vi "Content.vi"(7 "Context":refnum<class "Context.lvclass">, 8 "Error In":errorcluster, 11 "Tag In":refnum<class "Tag.lvclass">) -> (0 "Error Out":errorcluster, 2 "Content":string, 3 "Tag Out":refnum<class "Tag.lvclass">)   [LabVIEW 2018, in "Toolkit.lvlib" / "Nodes.lvlib" / "Tag.lvclass"]
uses:
  Tag.lvclass
  Support/Context/Context.lvclass
  Tag.lvclass/Tag.ctl
  Data/String/String.lvclass
  Data/String/String.lvclass/String.ctl
  Data/Abstract/Abstract.lvclass
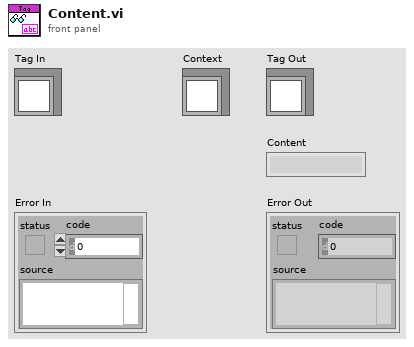
[diagram p1: front panel]
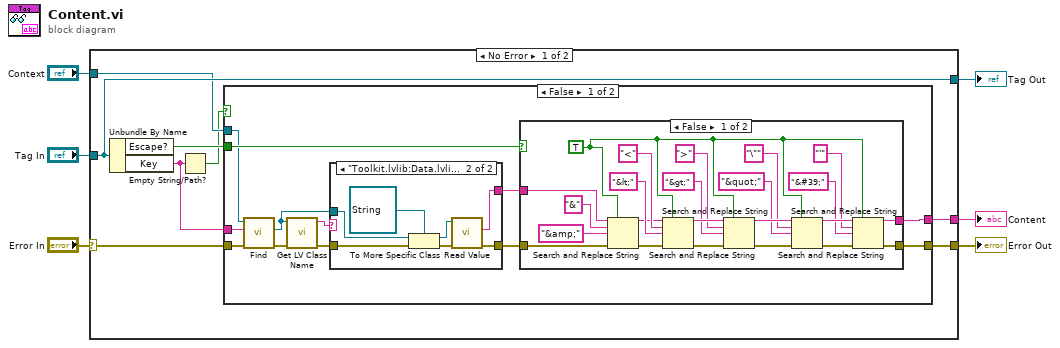
[diagram p0: block diagram]
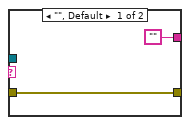
[diagram p2: hidden frame]
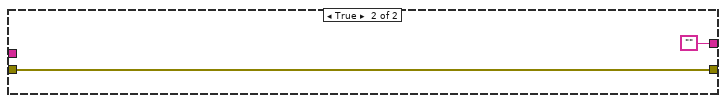
[diagram p4: hidden frame]
diagram:
  n1 = case shown="No Error" "Error In" {
    selector: "Error In" -> [w9 w63]
    tunnel: "Tag In" -> [w14 w64]
    tunnel: [w14 w64] -> w4
    tunnel: [w13 w63] -> w3
    tunnel: [w12 _] -> w2
    tunnel: "Context" -> [w10 _]
    frame No Error {
      n2 = Unbundle By Name(w14) -> ("Escape?"=w11:bool, "Key"=w8:string)
      n3 = Empty String/Path?(string/path=w8) -> (empty?=w7:bool)
      n4 = case shown="False" w7 {
        tunnel: [w26 w62] -> w13
        tunnel: [w25 ""] -> w12
        tunnel: w11 -> [w24 _]
        tunnel: w10 -> [w19 _]
        tunnel: w8 -> [w18 _]
        tunnel: w9 -> [w17 w62]
        frame False {
          n5 = call "Find.vi"("Error In"=w17, "Key"=w18, "Context In"=w19) -> ("Error Out"=w16:errorcluster, "Datum"=w15:refnum<class "Abstract.lvclass">)  [unwired: 5 in, 2 out]
          n6 = call <vilib>:"Get LV Class Name.vi"("error in (no error)"=w16, "object"=w15) -> ("error out"=w22:errorcluster, "class name"=w23:string)  [unwired: 8 in]
          n7 = case shown="\"Toolkit.lvlib:Data.lvlib:String.lvclass\"" w23 {
            tunnel: w22 -> [w28 w35]
            tunnel: w15 -> [_ w33]
            tunnel: [w28 w30] -> w21
            tunnel: ["" w29] -> w20
            frame "", Default {
            }
            frame "Toolkit.lvlib:Data.lvlib:String.lvclass" {
              n8 = To More Specific Class(target class=refnum<class "String.lvclass"> refnum ("Toolkit.lvlib:Data.lvlib:String.lvclass"), reference=w33, error in=w35) -> (specific class reference=w31:refnum<class "String.lvclass">, error out=w32:errorcluster)
              n9 = call "Read Value.vi"("Error In"=w32, "String In"=w31) -> ("Error Out"=w30:errorcluster, "Value"=w29:string)  [unwired: 7 in, 1 out]
            }
          }
          n10 = case shown="False" w24 {
            tunnel: [w39 w59] -> w26
            tunnel: [w38 w60] -> w25
            tunnel: w21 -> [w37 w59]
            tunnel: w20 -> [w36 w60]
            frame False {
              w42 = TRUE ("replace all? (F)")
              n11 = Search and Replace String(replace all?=w42, input string=w36, search string="&", replace string="&amp;" ("replace string (\"\")"), error in=w37) -> (result string=w54:string, error out=w53:errorcluster)  [unwired: 3 in, 2 out]
              n12 = Search and Replace String(replace all?=w42, input string=w54, search string="<", replace string="&lt;" ("replace string (\"\")"), error in=w53) -> (result string=w51:string, error out=w52:errorcluster)  [unwired: 3 in, 2 out]
              n13 = Search and Replace String(replace all?=w42, input string=w51, search string=">", replace string="&gt;" ("replace string (\"\")"), error in=w52) -> (result string=w47:string, error out=w48:errorcluster)  [unwired: 3 in, 2 out]
              n14 = Search and Replace String(replace all?=w42, input string=w47, search string="\"" ("replace string (\"\")"), replace string="&quot;" ("replace string (\"\")"), error in=w48) -> (result string=w44:string, error out=w43:errorcluster)  [unwired: 3 in, 2 out]
              n15 = Search and Replace String(replace all?=w42, input string=w44, search string="'", replace string="&#39;" ("replace string (\"\")"), error in=w43) -> (result string=w38:string, error out=w39:errorcluster)  [unwired: 3 in, 2 out]
            }
            frame True {
            }
          }
        }
        frame True {
        }
      }
    }
    frame Error {
    }
  }
  "Error Out" <- w3
  "Tag Out" <- w4
  "Content" <- w2
